vi "TimingFunctions_convertJavaToLvTimestamp.vi"(1 "TimeStamp (Java)":u64, 3 "TimeLimitation":T1 {"ToUTC" format="%^<%H:%M:%S%3u %p\n%d/%m/%Y>T"; "FromUTC" format="%^<%H:%M:%S%3u %p\n%d/%m/%Y>T"}) -> (15 "TimeStamp (LV) UTC":timestamp format="%^<%H:%M:%S%3u %p\n%d/%m/%Y>T")   [LabVIEW 2016]
doc: "Konvertiert einen Java Timestamp (startend am 1.1.1970, in 1/1000s Schritten, U64) in einen LabVIEW Timestamp\n\n15.05.14 / sige"
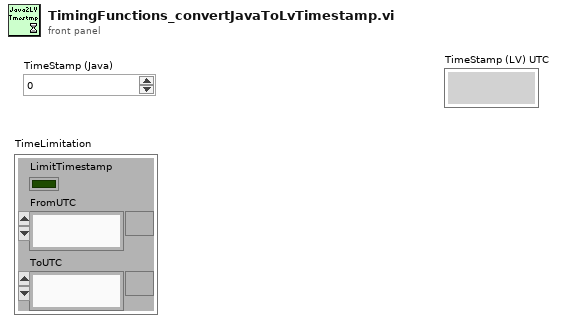
[diagram p1: front panel]
types:
  T1 = cluster{"LimitTimestamp":bool, "FromUTC":timestamp, "ToUTC":timestamp}
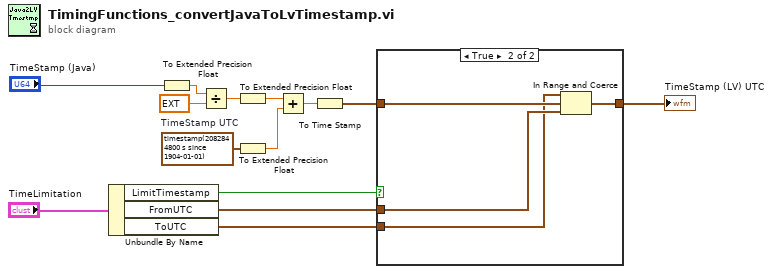
[diagram p0: block diagram]
diagram:
  w11 = timestamp(2082844800 s since 1904-01-01)  # TimeStamp UTC
  n1 = Unbundle By Name("TimeLimitation") -> ("LimitTimestamp"=w3:bool, "FromUTC"=w2:timestamp, "ToUTC"=w1:timestamp)
  n2 = To Extended Precision Float(1:"TimeStamp (Java)") -> (0:w9:ext)
  n3 = Divide(x=w9, y=ext 1000.0) -> (x/y=w10:ext)
  n4 = To Extended Precision Float(1:w10) -> (0:w14:ext)
  n5 = To Extended Precision Float(1:w11) -> (0:w12:ext)
  n6 = Add(x=w14, y=w12) -> (x+y=w7:ext)
  n7 = To Time Stamp(1:w7) -> (0:w6:timestamp)
  n8 = case shown="True" w3 {
    tunnel: w6 -> [w15 w19]
    tunnel: [w15 w18] -> w5
    tunnel: w2 -> [_ w17]
    tunnel: w1 -> [_ w16]
    frame False {
    }
    frame True {
      n9 = In Range and Coerce(upper limit=w16, x=w19, lower limit=w17) -> (coerced(x)=w18:timestamp)  [unwired: 1 out]
    }
  }
  "TimeStamp (LV) UTC" <- w5
